vi "ZC_pp_xh.vi"(0 "key":string, 6 "name":string, 7 "LabVIEW Web Service Request":refnum<class "Web Request.lvclass"> caption="LabVIEW Web服务请求", 8 "id":string, 9 "action":string, 10 "number":string, 11 "caozuo":string) -> (2 "error":errorcluster)   [LabVIEW 2017]
uses:
  <vilib>/wsapi/Web Request.lvclass
panel:
  out "postdata":string caption="post数据"
  out "error out":errorcluster caption="错误输出"
  # "Web服务请求输入接线端用于调用“Web服务”选板的VI。除非不需要访问该选板，否则不要在连线板上删除这个输入接线端。"
  # "添加至连线板的每一个其他输入控件，在URL中对应于一个输入。如需在接线端模式输出（默认设置）下包含显示控件，则该显示控件必须与连线板相连。"
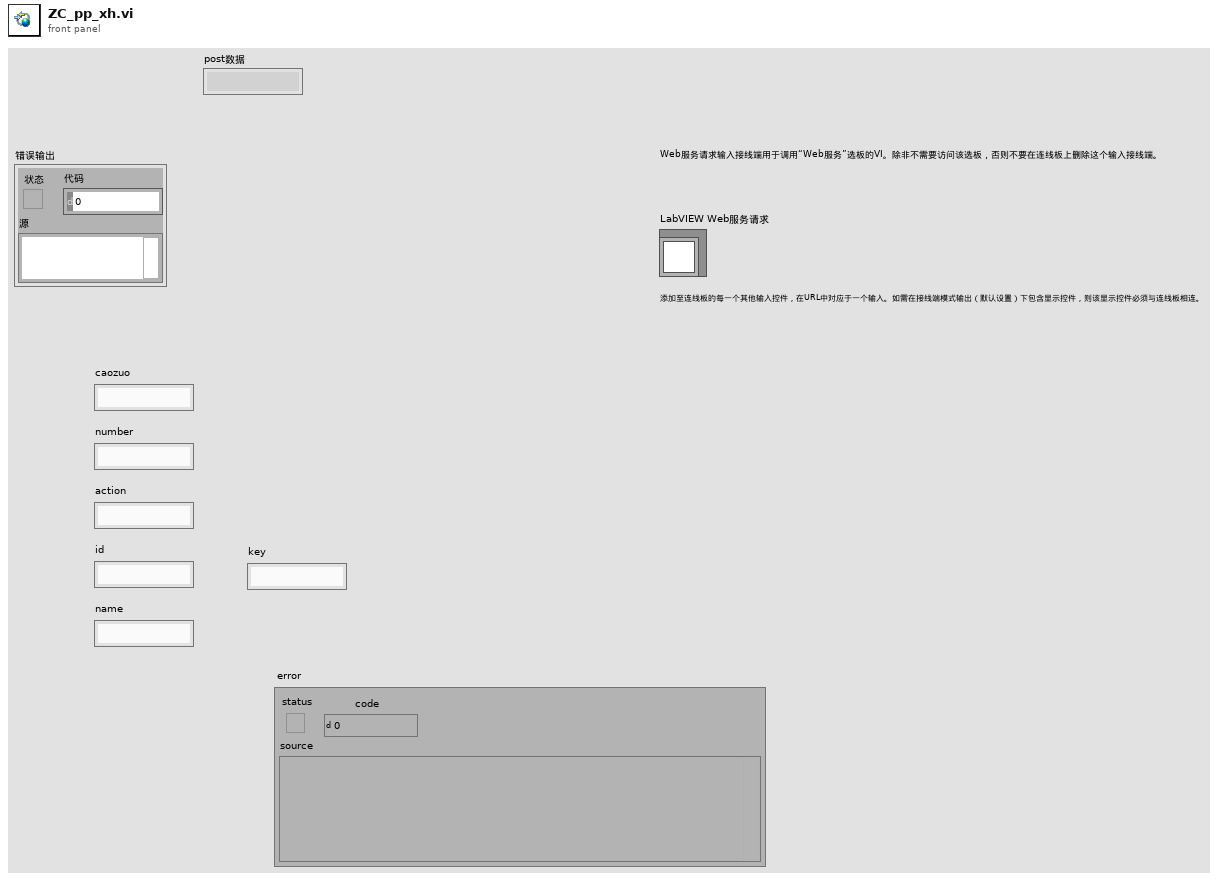
[diagram p1: front panel]
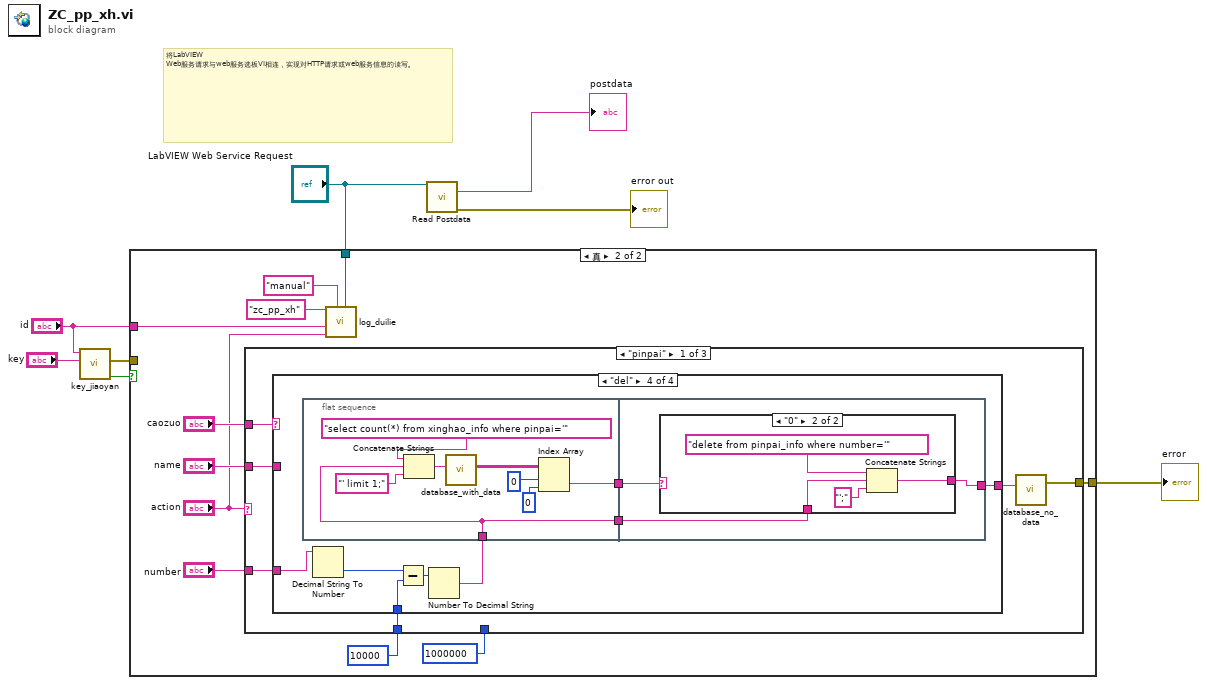
[diagram p0: block diagram]
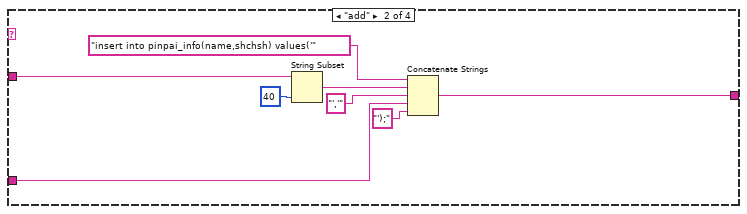
[diagram p4: hidden frame]
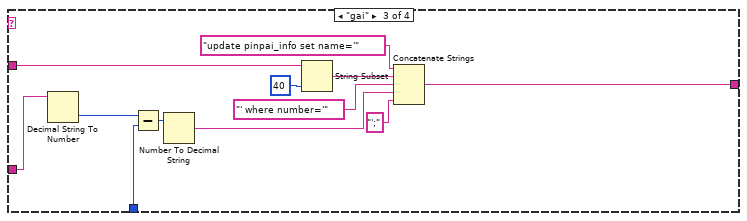
[diagram p5: hidden frame]
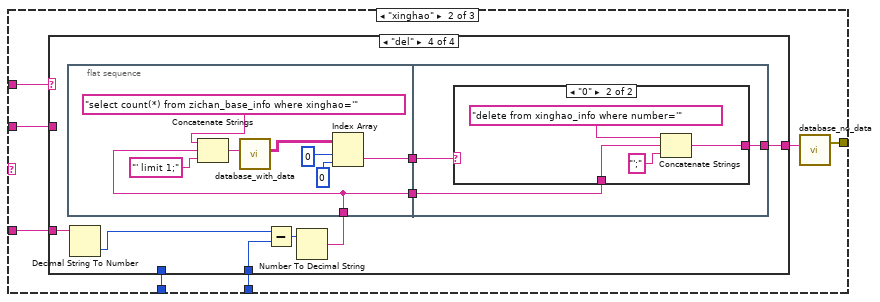
[diagram p7: hidden frame]
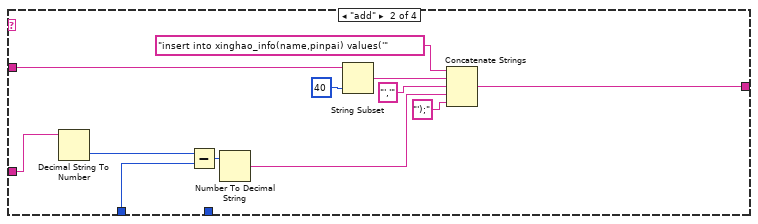
[diagram p9: hidden frame]
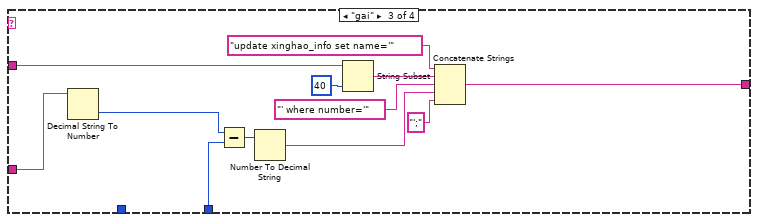
[diagram p10: hidden frame]
diagram:
  # "将LabVIEW Web服务请求与web服务选板VI相连，实现对HTTP请求或web服务信息的读写。"
  n1 = call "key_jiaoyan.vi"("key_client"="key", "gonghao"="id") -> ("jy"=w2:bool, "error"=w1:errorcluster)  [unwired: 8 in]
  n2 = case shown="真" w2 {
    tunnel: [w9 w20] -> w8
    tunnel: "LabVIEW Web Service Request" -> [_ w12]
    tunnel: "id" -> [_ w10]
    tunnel: w1 -> [w9 _]
    frame False {
    }
    frame True {
      n3 = case shown="\"pinpai\"" "action" {
        tunnel: [w25 w75 _] -> w20
        tunnel: "caozuo" -> [w24 w74 _]
        tunnel: "name" -> [w23 w73 _]
        tunnel: "number" -> [w22 w72 _]
        tunnel: 10000 ("y") -> [w21 w71 _]
        tunnel: 1000000 ("y") -> [_ w70 _]
        frame "pinpai" {
          n4 = case shown="\"del\"" w24 {
            tunnel: [_ w31 w42 w54] -> w26
            tunnel: w23 -> [_ w30 w41 _]
            tunnel: w22 -> [_ w27 w36 w49]
            tunnel: w21 -> [_ _ w35 w47]
            frame "假", Default {
            }
            frame "add" {
              n5 = String Subset(string=w30, length (rest)=40 ("长度（剩余）")) -> (substring=w33:string)  [unwired: 1 in]
              n6 = Concatenate Strings("insert into pinpai_info(name,shchsh) values('" ("格式字符串"), w33, "','" ("字符串"), w27, "');" ("字符串")) -> (w31:string)
            }
            frame "gai" {
              n7 = Decimal String To Number(string=w36) -> (number=w38:i32)  [unwired: 2 in, 1 out]
              n8 = Subtract(x=w38, y=w35) -> (x-y=w39:i32)
              n9 = Number To Decimal String(number=w39) -> (decimal integer string=w37:string)  [unwired: 1 in]
              n10 = String Subset(string=w41, length (rest)=40 ("长度（剩余）")) -> (substring=w45:string)  [unwired: 1 in]
              n11 = Concatenate Strings("update pinpai_info set name='" ("格式字符串"), w45, "' where number='" ("字符串"), w37, "';" ("字符串")) -> (w42:string)
            }
            frame "del" {
              n12 = flat-sequence {
                tunnel: w48 -> [w60]
                tunnel: [w60] -> w53
                tunnel: [w55] -> w52
                tunnel: [w65] -> w54
                tunnel: w53 -> [w64]
                tunnel: w52 -> [w63]
                frame #0 {
                  n13 = Concatenate Strings("select count(*) from xinghao_info where pinpai='" ("格式字符串"), w60, "' limit 1;" ("字符串")) -> (w59:string)
                  n14 = call "database_with_data.vi"("input"=w59) -> ("Data"=w56:string[][])  [unwired: 9 in, 1 out]
                  n15 = Index Array(array=w56, index (row)=0 ("索引 (行)"), index (col)=0 ("禁用的索引 (列)")) -> (element=w55:string)
                }
                frame #1 {
                  n16 = case shown="\"0\"" w63 {
                    tunnel: [_ w67] -> w65
                    tunnel: w64 -> [_ w66]
                    frame "假", Default {
                    }
                    frame "0" {
                      n17 = Concatenate Strings("delete from pinpai_info where number='" ("格式字符串"), w66, "';" ("字符串")) -> (w67:string)
                    }
                  }
                }
              }
              n18 = Decimal String To Number(string=w49) -> (number=w51:i32)  [unwired: 2 in, 1 out]
              n19 = Subtract(x=w51, y=w47) -> (x-y=w50:i32)
              n20 = Number To Decimal String(number=w50) -> (decimal integer string=w48:string)  [unwired: 1 in]
            }
          }
          n21 = call "database_no_data.vi"("input"=w26) -> ("error"=w25:errorcluster)  [unwired: 2 in]
        }
        frame "xinghao" {
          n22 = case shown="\"del\"" w74 {
            tunnel: [_ w85 w96 w102] -> w76
            tunnel: w73 -> [_ w84 w95 _]
            tunnel: w72 -> [_ w79 w93 w103]
            tunnel: w71 -> [_ w77 _ _]
            tunnel: w70 -> [_ _ w89 w101]
            frame "假", Default {
            }
            frame "add" {
              n23 = Decimal String To Number(string=w79) -> (number=w81:i32)  [unwired: 2 in, 1 out]
              n24 = Subtract(x=w81, y=w77) -> (x-y=w80:i32)
              n25 = Number To Decimal String(number=w80) -> (decimal integer string=w78:string)  [unwired: 1 in]
              n26 = String Subset(string=w84, length (rest)=40 ("长度（剩余）")) -> (substring=w87:string)  [unwired: 1 in]
              n27 = Concatenate Strings("insert into xinghao_info(name,pinpai) values('" ("格式字符串"), w87, "','" ("字符串"), w78, "');" ("字符串")) -> (w85:string)
            }
            frame "gai" {
              n28 = Decimal String To Number(string=w93) -> (number=w92:i32)  [unwired: 2 in, 1 out]
              n29 = Subtract(x=w92, y=w89) -> (x-y=w91:i32)
              n30 = Number To Decimal String(number=w91) -> (decimal integer string=w90:string)  [unwired: 1 in]
              n31 = String Subset(string=w95, length (rest)=40 ("长度（剩余）")) -> (substring=w99:string)  [unwired: 1 in]
              n32 = Concatenate Strings("update xinghao_info set name='" ("格式字符串"), w99, "' where number='" ("字符串"), w90, "';" ("字符串")) -> (w96:string)
            }
            frame "del" {
              n33 = flat-sequence {
                tunnel: w104 -> [w114]
                tunnel: [w114] -> w108
                tunnel: [w109] -> w107
                tunnel: [w119] -> w102
                tunnel: w108 -> [w118]
                tunnel: w107 -> [w117]
                frame #0 {
                  n34 = Concatenate Strings("select count(*) from zichan_base_info where xinghao='" ("格式字符串"), w114, "' limit 1;" ("字符串")) -> (w113:string)
                  n35 = call "database_with_data.vi"("input"=w113) -> ("Data"=w110:string[][])  [unwired: 9 in, 1 out]
                  n36 = Index Array(array=w110, index (row)=0 ("索引 (行)"), index (col)=0 ("禁用的索引 (列)")) -> (element=w109:string)
                }
                frame #1 {
                  n37 = case shown="\"0\"" w117 {
                    tunnel: [_ w121] -> w119
                    tunnel: w118 -> [_ w120]
                    frame "假", Default {
                    }
                    frame "0" {
                      n38 = Concatenate Strings("delete from xinghao_info where number='" ("格式字符串"), w120, "';" ("字符串")) -> (w121:string)
                    }
                  }
                }
              }
              n39 = Decimal String To Number(string=w103) -> (number=w106:i32)  [unwired: 2 in, 1 out]
              n40 = Subtract(x=w106, y=w101) -> (x-y=w105:i32)
              n41 = Number To Decimal String(number=w105) -> (decimal integer string=w104:string)  [unwired: 1 in]
            }
          }
          n42 = call "database_no_data.vi"("input"=w76) -> ("error"=w75:errorcluster)  [unwired: 2 in]
        }
        frame Default {
        }
      }
      n43 = call "log_duilie.vi"("LabVIEW Web Service Request"=w12, "type"="manual", "action"="action", "user"=w10, "yw"="zc_pp_xh") -> ()  [unwired: 7 in]
    }
  }
  "error" <- w8
  n44 = call <vilib>:"Read Postdata.vi"("LabVIEW Web Service Request"="LabVIEW Web Service Request") -> ("postdata"=→"postdata":string, "error out"=→"error out":errorcluster)  [unwired: 12 in, 1 out]
